vi "Solve_Correspond_Problem_based_on_Cost_F()-4.vi"(0 "[IN] Cost function":i8[](array[numeric]), 1 "[IN] Still connected\ntracks in group":T2, 3 "[IN] Subtracks":T3(array[cluster]), 7 "[IN] Index of Earliest \nProblem Point Inside":i32, 9 "[IN] # of Longest track\nInside the Tracks Group":i32, 11 "error IN":errorcluster, 13 "[IN] Special case!":bool) -> (4 "[OUT] Clusters for Re\nconstructed Tracks":T1, 15 "error OUT":errorcluster)   [LabVIEW 2013]
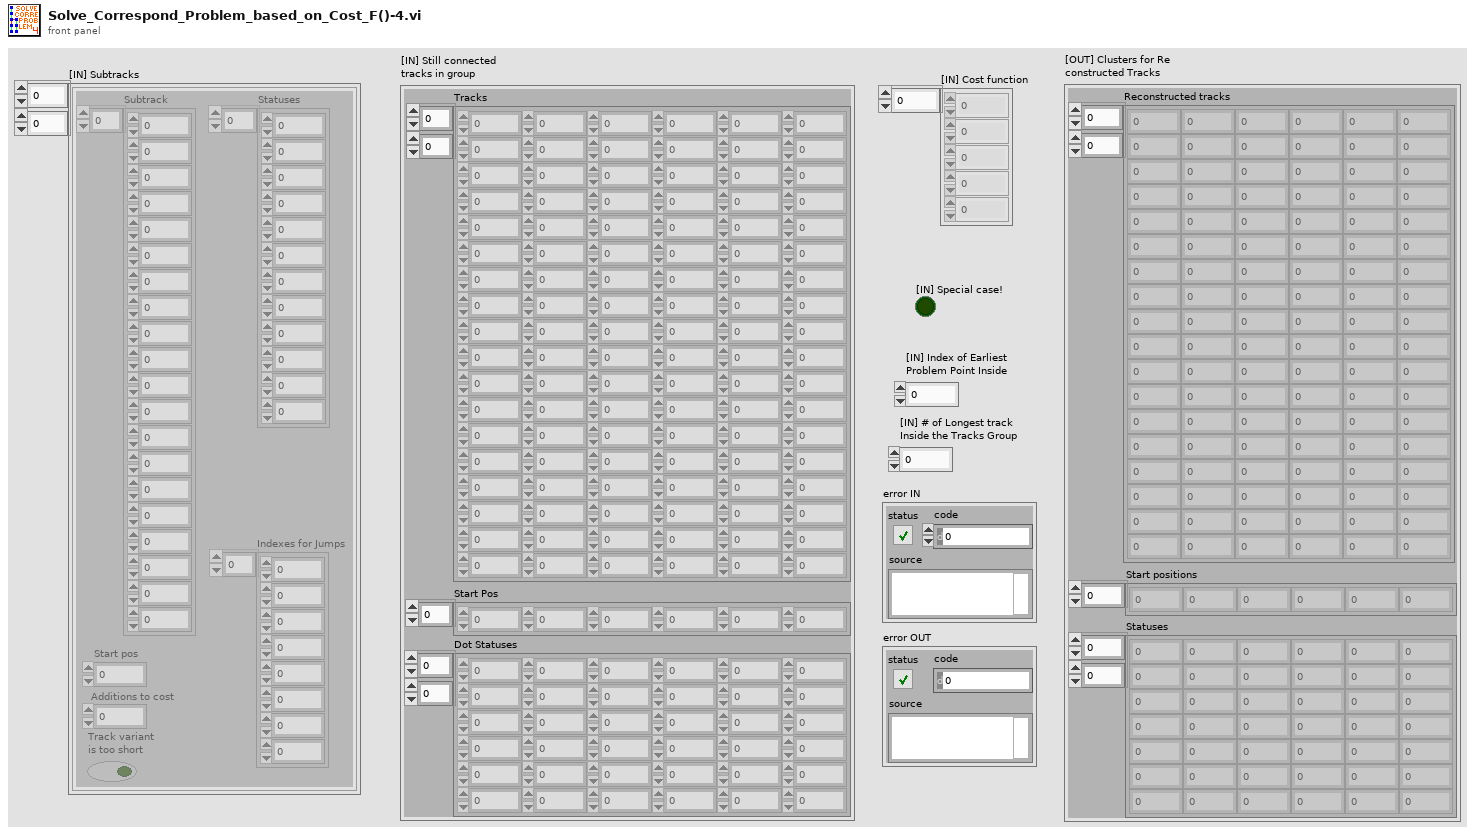
[diagram p1: front panel]
types:
  T1 = cluster{"Reconstructed tracks":dbl[][], "Start positions":i32[], "Statuses":i16[][]}
  T2 = cluster{"Tracks":dbl[][], "Start Pos":i32[], "Dot Statuses":i16[][]}
  T3 = cluster{"Subtrack":dbl[], "Statuses":i16[], "Start pos":i32, "Additions to cost":i32, "Track variant \nis too short":bool, "Indexes for Jumps":i32[]}[][]
  T4 = cluster{"Subtrack":dbl[], "Statuses":i16[], "Start pos":i32, "Additions to cost":i32, "Track variant \nis too short":bool, "Indexes for Jumps":i32[]}
  T5 = cluster{"Subtrack":dbl[], "Statuses":i16[], "Start pos":i32, "Additions to cost":i32, "Track variant \nis too short":bool, "Indexes for Jumps":i32[]}[]
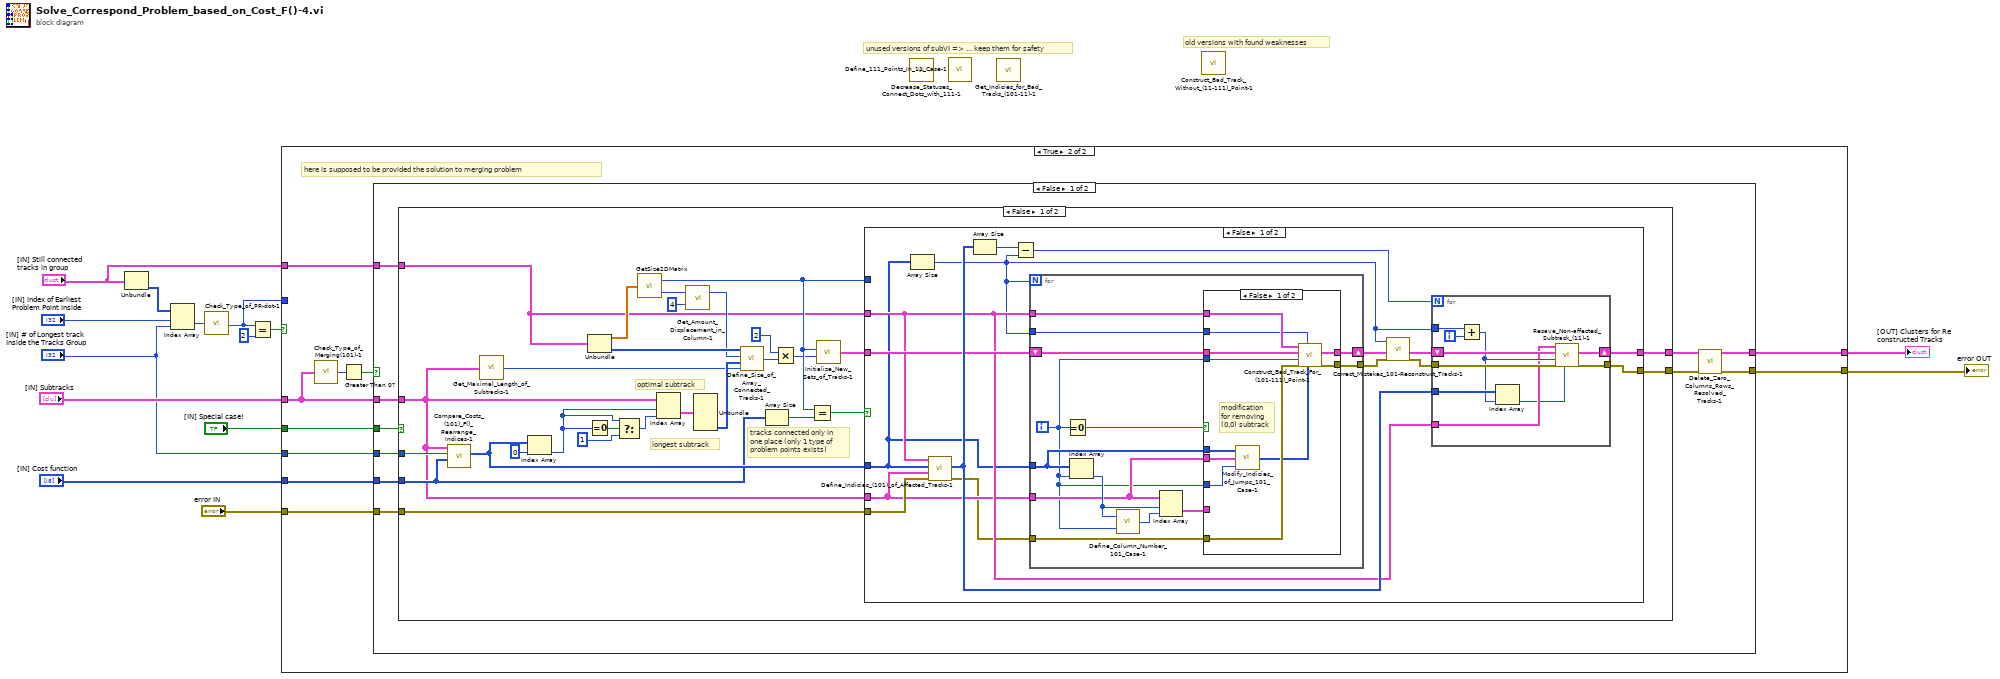
[diagram p0: block diagram]
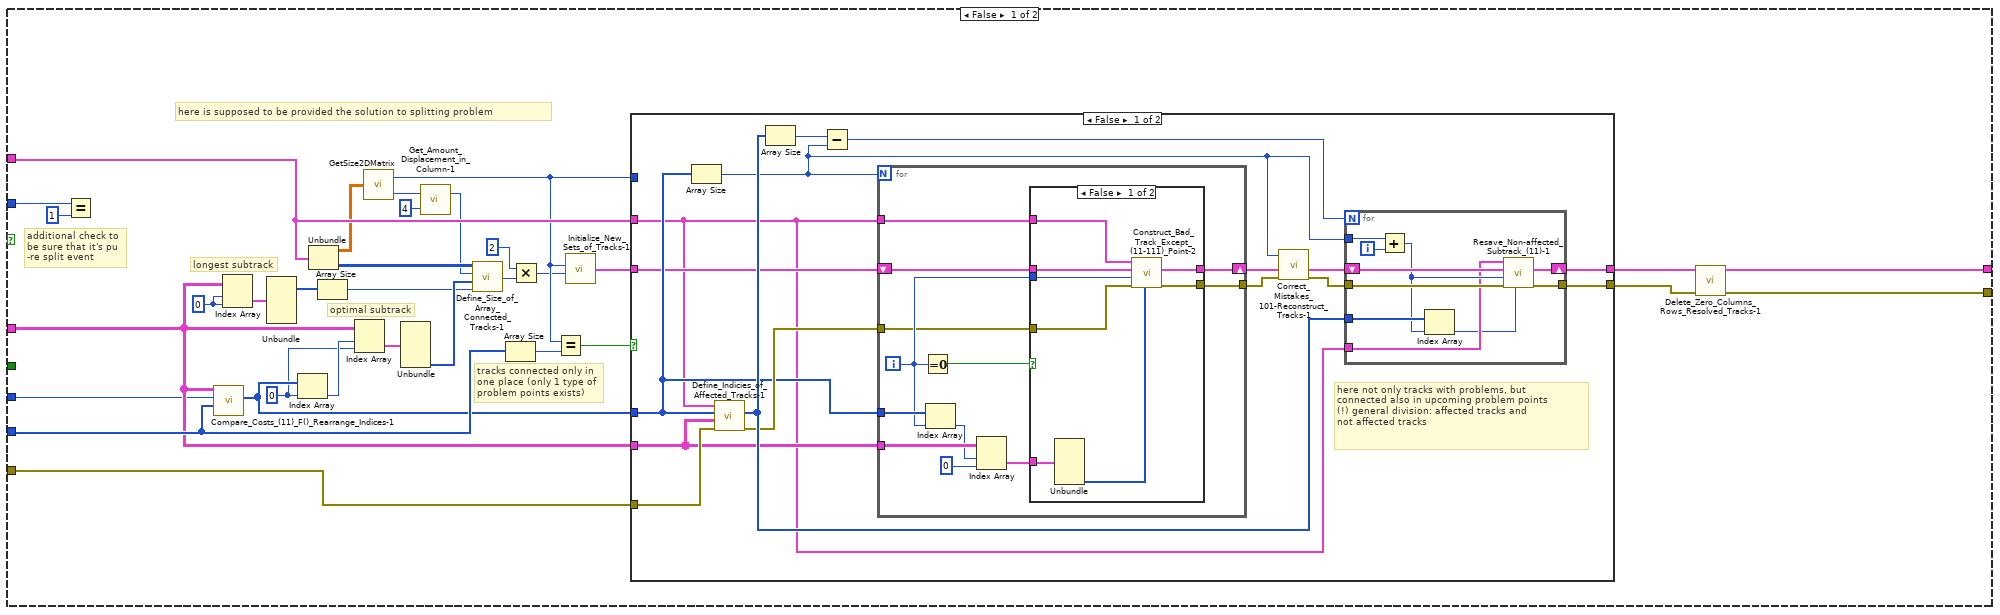
[diagram p2: hidden frame]
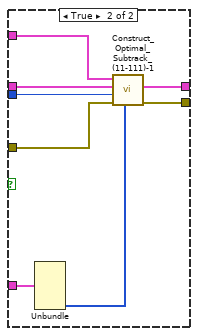
[diagram p3: hidden frame]
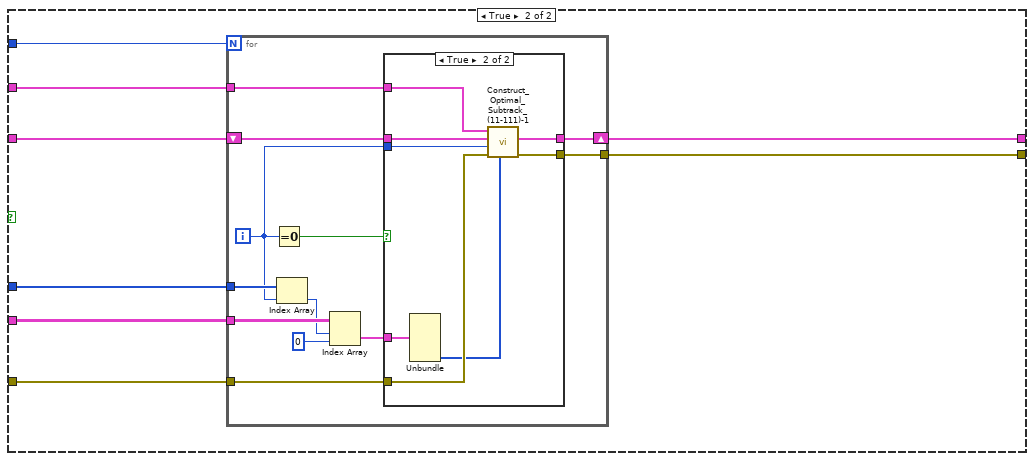
[diagram p4: hidden frame]
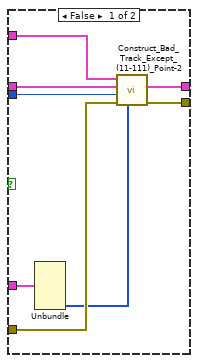
[diagram p5: hidden frame]
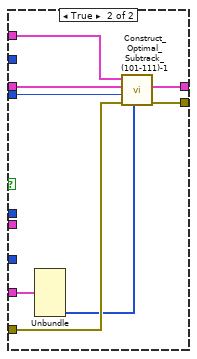
[diagram p6: hidden frame]
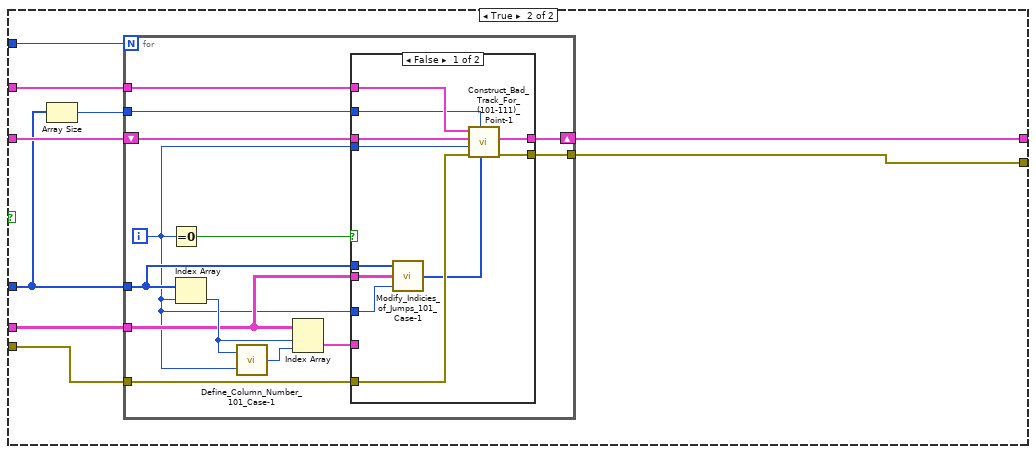
[diagram p7: hidden frame]
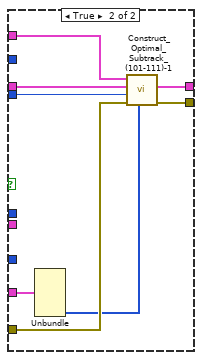
[diagram p8: hidden frame]
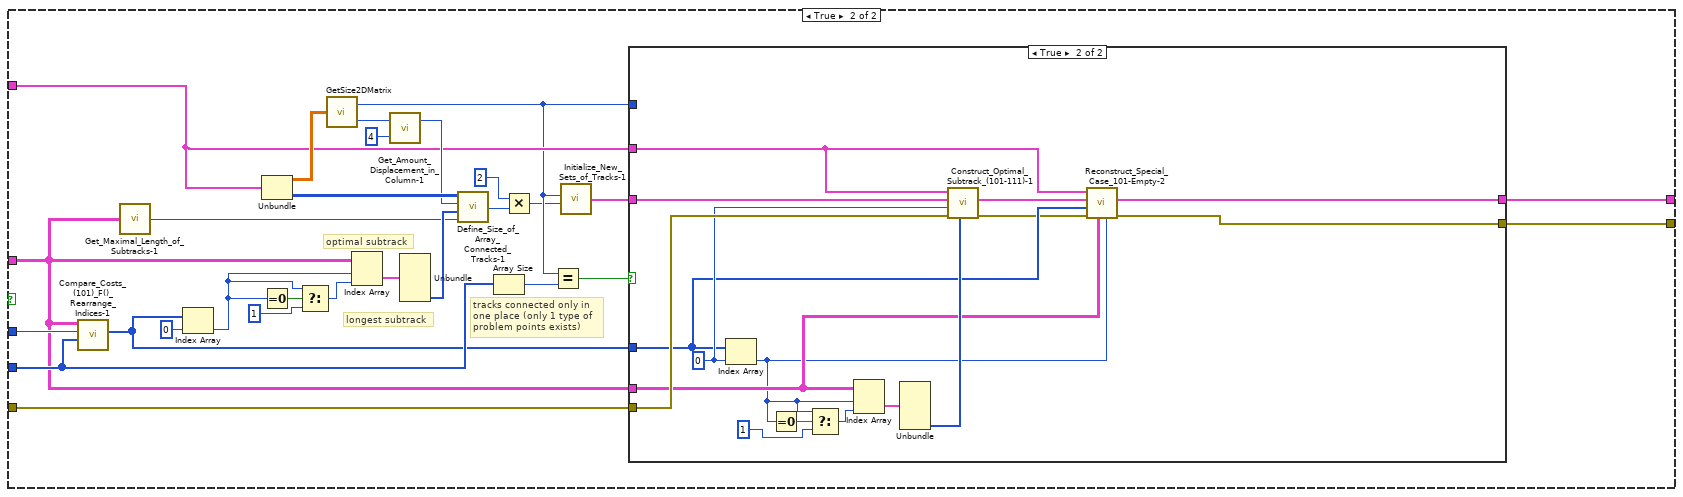
[diagram p9: hidden frame]
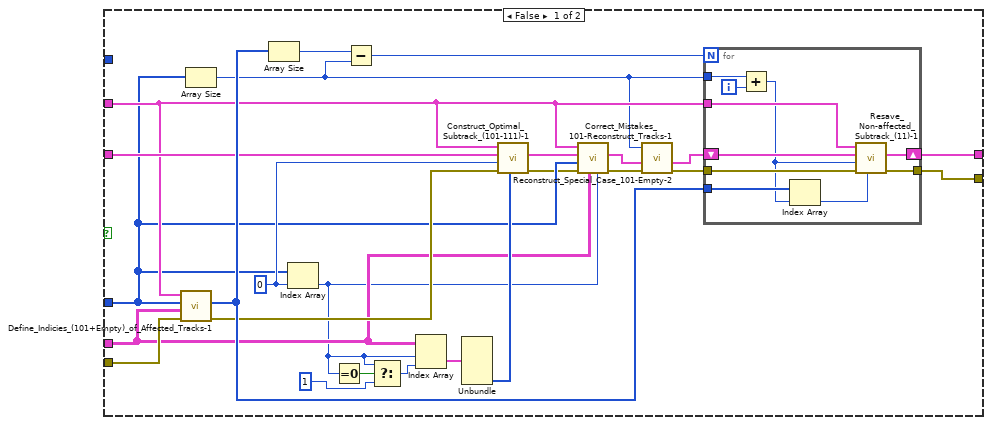
[diagram p10: hidden frame]
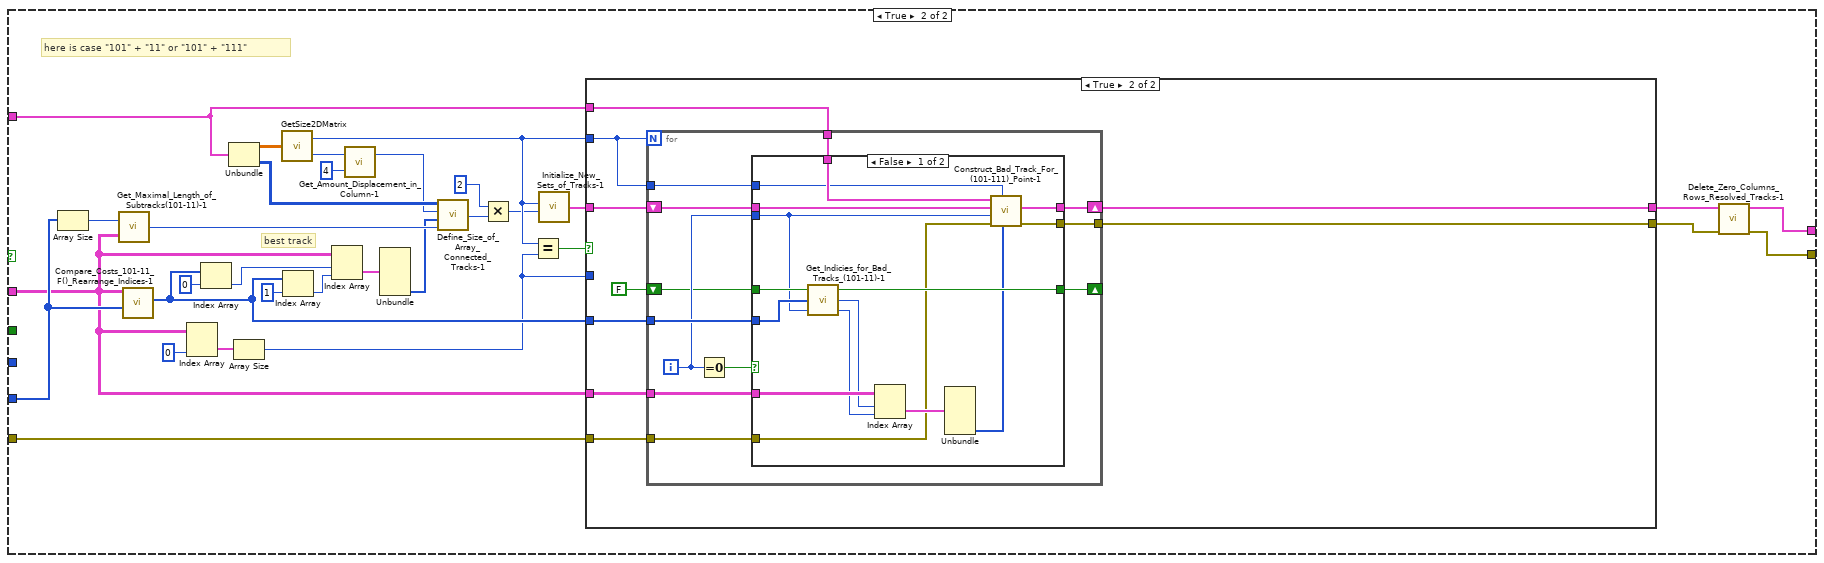
[diagram p11: hidden frame]
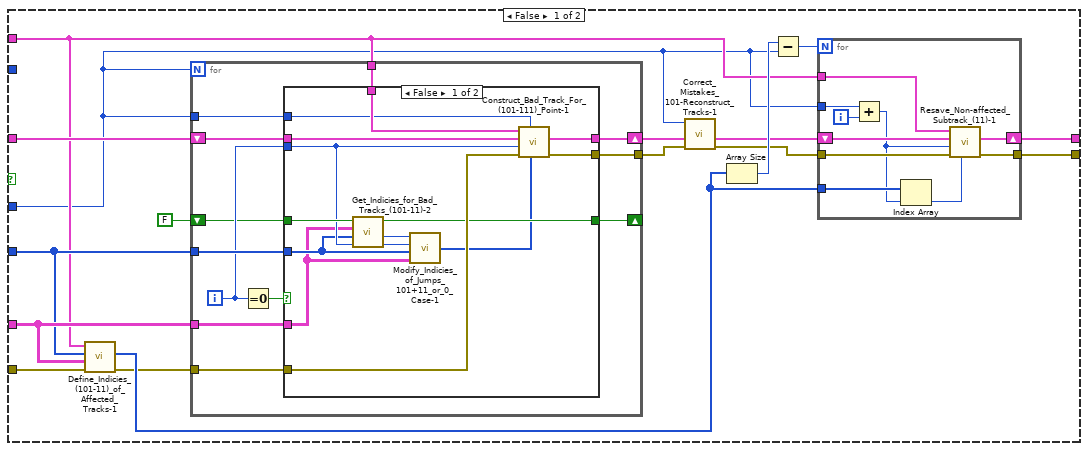
[diagram p12: hidden frame]
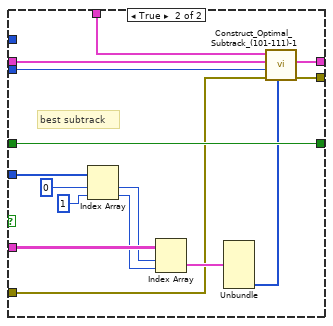
[diagram p13: hidden frame]
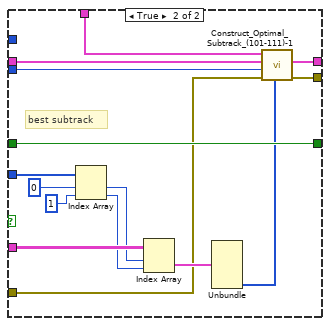
[diagram p14: hidden frame]
diagram:
  # "old versions with found weaknesses"
  # "unused versions of subVI => ... keep them for safety"
  n1 = Unbundle("[IN] Still connected\ntracks in group") -> ("Dot Statuses"=w13:i16[][])  [unwired: 2 out]
  n2 = Index Array(array=w13, index (row)="[IN] Index of Earliest \nProblem Point Inside", index (col)="[IN] # of Longest track\nInside the Tracks Group") -> (element=w12:i16)
  n3 = call "Check_Type_of_PR-dot-1.vi"("[IN] dot status"=w12) -> ("[OUT] Type of\nproblem dot"=w5:i32)
  n4 = Equal?(x=w5, y=2) -> (x = y?=w11:bool)
  n5 = case shown="True" w11 {
    tunnel: "[IN] Subtracks" -> [w45 w141]
    tunnel: "[IN] Still connected\ntracks in group" -> [w42 w145]
    tunnel: "error IN" -> [w40 w146]
    tunnel: "[IN] Cost function" -> [w46 w143]
    tunnel: w5 -> [w44 _]
    tunnel: "[IN] # of Longest track\nInside the Tracks Group" -> [w41 w144]
    tunnel: [w39 w139] -> w3
    tunnel: [w38 w138] -> w2
    tunnel: "[IN] Special case!" -> [_ w137]
    frame False {
      w23 = 0 ("index")
      w29 = 0 ("index")
      # "longest subtrack"
      # "tracks connected only in \none place (only 1 type of \nproblem points exists)"
      # "here is supposed to be provided the solution to splitting problem"
      # "optimal subtrack"
      # "additional check to \nbe sure that it's pu\n-re split event"
      n6 = Equal?(x=w44, y=1) -> ()  [unwired: 1 out]
      n7 = call "Compare_Costs_(11)_F()_Rearrange_Indices-1.vi"("[IN] Cost functions"=w46, "[IN] # of Longest track\nInside the Tracks Group"=w41, "[IN] Subtracks"=w45) -> ("[OUT] Indicies of sub\ntracks for transforma\ntion (resolving)"=w30:i32[])  [unwired: 4 in]
      n8 = Index Array(array=w45, index (row)=w23, index (col)=w23) -> (element=w22:T4)
      n9 = Unbundle(w22) -> ("Statuses"=w21:i16[])  [unwired: 5 out]
      n10 = Index Array(array=w30, index=w29) -> (element=w31:i32)
      n11 = Unbundle(w42) -> ("Tracks"=w34:dbl[][], "Dot Statuses"=w36:i16[][])  [unwired: 1 out]
      n12 = Array Size(array=w21) -> (size(s)=w20:i32)
      n13 = Index Array(array=w45, index (row)=w31, index (col)=w29) -> (element=w37:T4)
      n14 = call "GetSize2DMatrix.vi"("Array IN (2D)"=w34) -> ("# Cols"=w28:i32, "# Rows"=w26:i32)
      n15 = Unbundle(w37) -> ("Indexes for Jumps"=w35:i32[])  [unwired: 5 out]
      n16 = call "Get_Amount_Displacement_in_Column-1.vi"("multiplier"=4, "# Rows"=w26) -> ("Displ amount"=w24:i32)  [unwired: 1 out]
      n17 = call "Define_Size_of_Array_Connected_Tracks-1.vi"("[IN] Size of Longest Array\nbetween Subtracks (0,0)"=w20, "[IN] Indexes for Jumps"=w35, "[IN] Original Array Size"=w24, "[IN] Dot Statuses"=w36) -> ("[OUT] # of Eleme\nnts in new Track"=w17:i32)  [unwired: 2 in]
      n18 = Array Size(array=w46) -> (size(s)=w33:i32)
      n19 = Multiply(x=2, y=w17) -> (x*y=w16:i32)
      n20 = Equal?(x=w28, y=w33) -> (x = y?=w32:bool)
      n21 = call "Initialize_New_Sets_of_Tracks-1.vi"("[IN] # of Eleme\nnts in New Tracks"=w16, "[IN] # previously \nconnected tracks"=w28) -> ("[OUT] Clusters for Re\nconstructed Tracks"=w27:T1)  [unwired: 4 in]
      n22 = case shown="False" w32 {
        tunnel: w28 -> [_ w108]
        tunnel: w42 -> [w52 w103]
        tunnel: w30 -> [w54 w107]
        tunnel: w45 -> [w56 w102]
        tunnel: w27 -> [w53 w106]
        tunnel: w40 -> [w62 w101]
        tunnel: [w57 w104] -> w19
        tunnel: [w58 w105] -> w18
        frame False {
          # "here not only tracks with problems, but\nconnected also in upcoming problem points\n(!) general division: affected tracks and \nnot affected tracks"
          n23 = Array Size(array=w54) -> (size(s)=w50:i32)
          n24 = call "Define_Indicies_of_Affected_Tracks-1.vi"("error IN"=w62, "[IN] Subtracks"=w56, "[IN] Indicies of sub\ntracks for transforma\ntion (resolving)"=w54, "[IN] Still connected\ntracks in group"=w52) -> ("error OUT"=w55:errorcluster, "[OUT] Indicies for Tr-\nack Reconstruction"=w59:i32[])  [unwired: 2 in]
          n25 = Array Size(array=w59) -> (size(s)=w61:i32)
          n26 = Subtract(x=w61, y=w50) -> (x-y=w60:i32)
          n27 = for {
            N: w50 -> [_]
            tunnel: w52 -> [w68]
            tunnel: w54 -> [w73]
            tunnel: w56 -> [w72]
            shift-right: [w65] -> w51
            shift-left: w53 -> [w67]
            tunnel: [w64] -> w48
            tunnel: w55 -> [w63]
            i -> [w66]
            n28 = Equal To 0?(x=w66) -> (x = 0?=w74:bool)
            n29 = Index Array(array=w73, index=w66) -> (element=w71:i32)
            n30 = Index Array(array=w72, index (row)=w71, index (col)=0 ("disabled index (col)")) -> (element=w69:T4)
            n31 = case shown="False" w74 {
              tunnel: w69 -> [w82 w90]
              tunnel: w68 -> [w81 w89]
              tunnel: w67 -> [w80 w87]
              tunnel: w66 -> [w79 w86]
              tunnel: [w75 w84] -> w65
              tunnel: w63 -> [w78 w88]
              tunnel: [w76 w83] -> w64
              frame False {
                n32 = Unbundle(w82) -> ("Indexes for Jumps"=w77:i32[])  [unwired: 5 out]
                n33 = call "Construct_Bad_Track_Except_(11-111)_Point-2.vi"("[IN] Indexes for Jumps"=w77, "error IN"=w78, "[IN] Index of recon\nstructed tracks"=w79, "[IN] Clusters for Re\nconstructed Tracks"=w80, "[IN] Still connected\ntracks in group"=w81) -> ("error OUT"=w76:errorcluster, "[OUT] Clusters for Re\nconstructed Tracks"=w75:T1)  [unwired: 5 in]
              }
              frame True {
                n34 = Unbundle(w90) -> ("Indexes for Jumps"=w85:i32[])  [unwired: 5 out]
                n35 = call "Construct_Optimal_Subtrack_(11-111)-1.vi"("[IN] Indexes for Jumps"=w85, "error IN"=w88, "[IN] Index of recon\nstructed tracks"=w86, "[IN] Clusters for Re\nconstructed Tracks"=w87, "[IN] Still connected\ntracks in group"=w89) -> ("error OUT"=w83:errorcluster, "[OUT] Clusters for Re\nconstructed Tracks"=w84:T1)  [unwired: 5 in]
              }
            }
          }
          n36 = call "Correct_Mistakes_101-Reconstruct_Tracks-1.vi"("error IN"=w48, "[IN] Clusters for Re\nconstructed Tracks"=w51, "[IN] Number of Subtracks"=w50) -> ("error OUT"=w47:errorcluster, "[OUT] Clusters for Re\nconstructed Tracks"=w49:T1)  [unwired: 3 in]
          n37 = for {
            N: w60 -> [_]
            tunnel: w47 -> [w96]
            tunnel: w59 -> [w100]
            tunnel: w50 -> [w98]
            tunnel: w52 -> [w94]
            shift-right: [w92] -> w57
            shift-left: w49 -> [w97]
            tunnel: [w91] -> w58
            i -> [w99]
            n38 = Add(x=w98, y=w99) -> (x+y=w95:i32)
            n39 = Index Array(array=w100, index=w95) -> (element=w93:i32)
            n40 = call "Resave_Non-affected_Subtrack_(11)-1.vi"("[IN] Index for Not\nAffected Track"=w93, "error IN"=w96, "[IN] Index of recon\nstructed tracks"=w95, "[IN] Clusters for Re\nconstructed Tracks"=w97, "[IN] Still connected\ntracks in group"=w94) -> ("error OUT"=w91:errorcluster, "[OUT] Clusters for Re\nconstructed Tracks"=w92:T1)  [unwired: 5 in]
          }
        }
        frame True {
          n41 = for {
            N: w108 -> [_]
            tunnel: w103 -> [w114]
            tunnel: w107 -> [w119]
            tunnel: w102 -> [w118]
            shift-right: [w111] -> w104
            shift-left: w106 -> [w113]
            tunnel: w101 -> [w110]
            tunnel: [w109] -> w105
            i -> [w112]
            n42 = Equal To 0?(x=w112) -> (x = 0?=w120:bool)
            n43 = Index Array(array=w119, index=w112) -> (element=w117:i32)
            n44 = Index Array(array=w118, index (row)=w117, index (col)=0 ("disabled index (col)")) -> (element=w115:T4)
            n45 = case shown="True" w120 {
              tunnel: w115 -> [w128 w136]
              tunnel: w114 -> [w127 w135]
              tunnel: w113 -> [w126 w133]
              tunnel: w112 -> [w125 w132]
              tunnel: [w122 w130] -> w111
              tunnel: w110 -> [w124 w134]
              tunnel: [w121 w129] -> w109
              frame False {
                n46 = Unbundle(w128) -> ("Indexes for Jumps"=w123:i32[])  [unwired: 5 out]
                n47 = call "Construct_Bad_Track_Except_(11-111)_Point-2.vi"("[IN] Indexes for Jumps"=w123, "error IN"=w124, "[IN] Index of recon\nstructed tracks"=w125, "[IN] Clusters for Re\nconstructed Tracks"=w126, "[IN] Still connected\ntracks in group"=w127) -> ("error OUT"=w121:errorcluster, "[OUT] Clusters for Re\nconstructed Tracks"=w122:T1)  [unwired: 5 in]
              }
              frame True {
                n48 = Unbundle(w136) -> ("Indexes for Jumps"=w131:i32[])  [unwired: 5 out]
                n49 = call "Construct_Optimal_Subtrack_(11-111)-1.vi"("[IN] Indexes for Jumps"=w131, "error IN"=w134, "[IN] Index of recon\nstructed tracks"=w132, "[IN] Clusters for Re\nconstructed Tracks"=w133, "[IN] Still connected\ntracks in group"=w135) -> ("error OUT"=w129:errorcluster, "[OUT] Clusters for Re\nconstructed Tracks"=w130:T1)  [unwired: 5 in]
              }
            }
          }
        }
      }
      n50 = call "Delete_Zero_Columns_Rows_Resolved_Tracks-1.vi"("error IN"=w18, "[IN] Clusters for Re\nconstructed Tracks"=w19) -> ("error OUT"=w38:errorcluster, "[OUT] Clusters for Re\nconstructed Tracks"=w39:T1)  [unwired: 4 in]
    }
    frame True {
      # "here is supposed to be provided the solution to merging problem"
      n51 = call "Check_Type_of_Merging(101)-1.vi"("[IN] Subtracks"=w141) -> ("[OUT] # of Additional Costs"=w142:i32)
      n52 = Greater Than 0?(x=w142) -> (x > 0?=w140:bool)
      n53 = case shown="False" w140 {
        tunnel: w146 -> [w156 w372]
        tunnel: w145 -> [w155 w371]
        tunnel: w144 -> [w154 _]
        tunnel: w143 -> [w151 w393]
        tunnel: w141 -> [w150 w373]
        tunnel: [w153 w367] -> w139
        tunnel: [w152 w366] -> w138
        tunnel: w137 -> [w147 _]
        frame False {
          n54 = case shown="False" w147 {
            tunnel: w156 -> [w173 w288]
            tunnel: w155 -> [w172 w292]
            tunnel: w154 -> [w170 w297]
            tunnel: w151 -> [w163 w296]
            tunnel: w150 -> [w162 w287]
            tunnel: [w161 w295] -> w149
            tunnel: [w160 w294] -> w148
            frame False {
              # "longest subtrack"
              # "tracks connected only in \none place (only 1 type of \nproblem points exists)"
              # "optimal subtrack"
              n55 = call "Compare_Costs_(101)_F()_Rearrange_Indices-1.vi"("[IN] Cost functions"=w163, "[IN] # of Longest track\nInside the Tracks Group"=w170, "[IN] Subtracks"=w162) -> ("[OUT] Indicies of sub\ntracks for transforma\ntion (resolving)"=w169:i32[])  [unwired: 4 in]
              n56 = call "Get_Maximal_Length_of_Subtracks-1.vi"("[IN] Subtracks"=w162) -> ("[OUT] Maximal Length"=w171:i32)
              n57 = Index Array(array=w169, index=0) -> (element=w165:i32)
              n58 = Unbundle(w172) -> ("Tracks"=w181:dbl[][], "Dot Statuses"=w183:i16[][])  [unwired: 1 out]
              n59 = Equal To 0?(x=w165) -> (x = 0?=w167:bool)
              n60 = Select(t=w165, s=w167, f=1) -> (s? t:f=w164:i32)
              n61 = call "GetSize2DMatrix.vi"("Array IN (2D)"=w181) -> ("# Cols"=w178:i32, "# Rows"=w176:i32)
              n62 = Index Array(array=w162, index (row)=w165, index (col)=w164) -> (element=w184:T4)
              n63 = call "Get_Amount_Displacement_in_Column-1.vi"("multiplier"=4, "# Rows"=w176) -> ("Displ amount"=w174:i32)  [unwired: 1 out]
              n64 = Unbundle(w184) -> ("Indexes for Jumps"=w182:i32[])  [unwired: 5 out]
              n65 = call "Define_Size_of_Array_Connected_Tracks-1.vi"("[IN] Size of Longest Array\nbetween Subtracks (0,0)"=w171, "[IN] Indexes for Jumps"=w182, "[IN] Original Array Size"=w174, "[IN] Dot Statuses"=w183) -> ("[OUT] # of Eleme\nnts in new Track"=w159:i32)  [unwired: 2 in]
              n66 = Array Size(array=w163) -> (size(s)=w180:i32)
              n67 = Multiply(x=2, y=w159) -> (x*y=w157:i32)
              n68 = Equal?(x=w178, y=w180) -> (x = y?=w179:bool)
              n69 = call "Initialize_New_Sets_of_Tracks-1.vi"("[IN] # of Eleme\nnts in New Tracks"=w157, "[IN] # previously \nconnected tracks"=w178) -> ("[OUT] Clusters for Re\nconstructed Tracks"=w177:T1)  [unwired: 4 in]
              n70 = case shown="False" w179 {
                tunnel: w178 -> [_ w251]
                tunnel: w172 -> [w195 w250]
                tunnel: w169 -> [w192 w246]
                tunnel: w162 -> [w194 w249]
                tunnel: w177 -> [w196 w247]
                tunnel: w173 -> [w198 w248]
                tunnel: [w190 w244] -> w161
                tunnel: [w191 w243] -> w160
                frame False {
                  n71 = Array Size(array=w192) -> (size(s)=w185:i32)
                  n72 = call "Define_Indicies_(101)_of_Affected_Tracks-1.vi"("error IN"=w198, "[IN] Subtracks"=w194, "[IN] Indicies of sub\ntracks for transforma\ntion (resolving)"=w192, "[IN] Still connected\ntracks in group"=w195) -> ("error OUT"=w193:errorcluster, "[OUT] Indicies for Tr-\nack Reconstruction"=w197:i32[])  [unwired: 2 in]
                  n73 = Array Size(array=w197) -> (size(s)=w200:i32)
                  n74 = Subtract(x=w200, y=w185) -> (x-y=w199:i32)
                  n75 = for {
                    N: w185 -> [_]
                    tunnel: w195 -> [w211]
                    tunnel: w192 -> [w203]
                    tunnel: w194 -> [w202]
                    tunnel: w193 -> [w210]
                    shift-right: [w208] -> w189
                    shift-left: w196 -> [w209]
                    tunnel: [w207] -> w187
                    tunnel: w185 -> [w206]
                    i -> [w201]
                    n76 = Equal To 0?(x=w201) -> (x = 0?=w213:bool)
                    n77 = Index Array(array=w203, index=w201) -> (element=w205:i32)
                    n78 = call "Define_Column_Number_101_Case-1.vi"("[IN] Current index"=w201, "[IN] Index of \nSubtrack Row"=w205) -> ("[OUT] Column for subtrack"=w204:i32)
                    n79 = Index Array(array=w202, index (row)=w205, index (col)=w204) -> (element=w212:T4)
                    n80 = case shown="False" w213 {
                      tunnel: w212 -> [_ w232]
                      tunnel: w211 -> [w221 w231]
                      tunnel: w201 -> [w218 w229]
                      tunnel: w210 -> [w217 w228]
                      tunnel: w209 -> [w219 w230]
                      tunnel: [w214 w225] -> w208
                      tunnel: [w215 w226] -> w207
                      tunnel: w206 -> [w220 _]
                      tunnel: w203 -> [w224 _]
                      tunnel: w202 -> [w223 _]
                      tunnel: w201 -> [w222 _]
                      frame False {
                        # "modification\nfor removing\n(0,0) subtrack"
                        n81 = call "Modify_Indicies_of_Jumps_101_Case-1.vi"("[IN] Current Index"=w222, "[IN] Subtracks"=w223, "[IN] Indicies of sub\ntracks for transforma\ntion (resolving)"=w224) -> ("[OUT] Indicies of Jumps"=w216:i32[])  [unwired: 2 in]
                        n82 = call "Construct_Bad_Track_For_(101-111)_Point-1.vi"("[IN] Indexes for Jumps"=w216, "[IN] Number of Co\nnnected Points"=w220, "error IN"=w217, "[IN] Index of recon\nstructed tracks"=w218, "[IN] Clusters for Re\nconstructed Tracks"=w219, "[IN] Still connected\ntracks in group"=w221) -> ("error OUT"=w215:errorcluster, "[OUT] Clusters for Re\nconstructed Tracks"=w214:T1)  [unwired: 4 in]
                      }
                      frame True {
                        n83 = Unbundle(w232) -> ("Indexes for Jumps"=w227:i32[])  [unwired: 5 out]
                        n84 = call "Construct_Optimal_Subtrack_(101-111)-1.vi"("[IN] Indexes for Jumps"=w227, "error IN"=w228, "[IN] Index of recon\nstructed tracks"=w229, "[IN] Clusters for Re\nconstructed Tracks"=w230, "[IN] Still connected\ntracks in group"=w231) -> ("error OUT"=w226:errorcluster, "[OUT] Clusters for Re\nconstructed Tracks"=w225:T1)  [unwired: 5 in]
                      }
                    }
                  }
                  n85 = call "Correct_Mistakes_101-Reconstruct_Tracks-1.vi"("error IN"=w187, "[IN] Clusters for Re\nconstructed Tracks"=w189, "[IN] Number of Subtracks"=w185) -> ("error OUT"=w186:errorcluster, "[OUT] Clusters for Re\nconstructed Tracks"=w188:T1)  [unwired: 3 in]
                  n86 = for {
                    N: w199 -> [_]
                    tunnel: w186 -> [w238]
                    tunnel: w197 -> [w242]
                    tunnel: w185 -> [w240]
                    tunnel: w195 -> [w236]
                    shift-right: [w234] -> w190
                    shift-left: w188 -> [w239]
                    tunnel: [w233] -> w191
                    i -> [w241]
                    n87 = Add(x=w240, y=w241) -> (x+y=w237:i32)
                    n88 = Index Array(array=w242, index=w237) -> (element=w235:i32)
                    n89 = call "Resave_Non-affected_Subtrack_(11)-1.vi"("[IN] Index for Not\nAffected Track"=w235, "error IN"=w238, "[IN] Index of recon\nstructed tracks"=w237, "[IN] Clusters for Re\nconstructed Tracks"=w239, "[IN] Still connected\ntracks in group"=w236) -> ("error OUT"=w233:errorcluster, "[OUT] Clusters for Re\nconstructed Tracks"=w234:T1)  [unwired: 5 in]
                  }
                }
                frame True {
                  n90 = Array Size(array=w246) -> (size(s)=w245:i32)
                  n91 = for {
                    N: w251 -> [_]
                    tunnel: w250 -> [w262]
                    tunnel: w246 -> [w254]
                    tunnel: w249 -> [w253]
                    tunnel: w248 -> [w261]
                    shift-right: [w259] -> w244
                    shift-left: w247 -> [w260]
                    tunnel: [w258] -> w243
                    tunnel: w245 -> [w257]
                    i -> [w252]
                    n92 = Equal To 0?(x=w252) -> (x = 0?=w264:bool)
                    n93 = Index Array(array=w254, index=w252) -> (element=w256:i32)
                    n94 = call "Define_Column_Number_101_Case-1.vi"("[IN] Current index"=w252, "[IN] Index of \nSubtrack Row"=w256) -> ("[OUT] Column for subtrack"=w255:i32)
                    n95 = Index Array(array=w253, index (row)=w256, index (col)=w255) -> (element=w263:T4)
                    n96 = case shown="False" w264 {
                      tunnel: w263 -> [_ w283]
                      tunnel: w262 -> [w272 w279]
                      tunnel: w252 -> [w268 w280]
                      tunnel: w261 -> [w267 w282]
                      tunnel: w260 -> [w270 w281]
                      tunnel: [w269 w278] -> w259
                      tunnel: [w266 w276] -> w258
                      tunnel: w257 -> [w271 _]
                      tunnel: w254 -> [w275 _]
                      tunnel: w253 -> [w274 _]
                      tunnel: w252 -> [w273 _]
                      frame False {
                        n97 = call "Modify_Indicies_of_Jumps_101_Case-1.vi"("[IN] Current Index"=w273, "[IN] Subtracks"=w274, "[IN] Indicies of sub\ntracks for transforma\ntion (resolving)"=w275) -> ("[OUT] Indicies of Jumps"=w265:i32[])  [unwired: 2 in]
                        n98 = call "Construct_Bad_Track_For_(101-111)_Point-1.vi"("[IN] Indexes for Jumps"=w265, "[IN] Number of Co\nnnected Points"=w271, "error IN"=w267, "[IN] Index of recon\nstructed tracks"=w268, "[IN] Clusters for Re\nconstructed Tracks"=w270, "[IN] Still connected\ntracks in group"=w272) -> ("error OUT"=w266:errorcluster, "[OUT] Clusters for Re\nconstructed Tracks"=w269:T1)  [unwired: 4 in]
                      }
                      frame True {
                        n99 = Unbundle(w283) -> ("Indexes for Jumps"=w277:i32[])  [unwired: 5 out]
                        n100 = call "Construct_Optimal_Subtrack_(101-111)-1.vi"("[IN] Indexes for Jumps"=w277, "error IN"=w282, "[IN] Index of recon\nstructed tracks"=w280, "[IN] Clusters for Re\nconstructed Tracks"=w281, "[IN] Still connected\ntracks in group"=w279) -> ("error OUT"=w276:errorcluster, "[OUT] Clusters for Re\nconstructed Tracks"=w278:T1)  [unwired: 5 in]
                      }
                    }
                  }
                }
              }
            }
            frame True {
              # "longest subtrack"
              # "tracks connected only in \none place (only 1 type of \nproblem points exists)"
              # "optimal subtrack"
              n101 = call "Compare_Costs_(101)_F()_Rearrange_Indices-1.vi"("[IN] Cost functions"=w296, "[IN] # of Longest track\nInside the Tracks Group"=w297, "[IN] Subtracks"=w287) -> ("[OUT] Indicies of sub\ntracks for transforma\ntion (resolving)"=w289:i32[])  [unwired: 4 in]
              n102 = call "Get_Maximal_Length_of_Subtracks-1.vi"("[IN] Subtracks"=w287) -> ("[OUT] Maximal Length"=w303:i32)
              n103 = Index Array(array=w289, index=0) -> (element=w299:i32)
              n104 = Unbundle(w292) -> ("Tracks"=w308:dbl[][], "Dot Statuses"=w310:i16[][])  [unwired: 1 out]
              n105 = Equal To 0?(x=w299) -> (x = 0?=w301:bool)
              n106 = Select(t=w299, s=w301, f=1) -> (s? t:f=w298:i32)
              n107 = call "GetSize2DMatrix.vi"("Array IN (2D)"=w308) -> ("# Cols"=w291:i32, "# Rows"=w306:i32)
              n108 = Index Array(array=w287, index (row)=w299, index (col)=w298) -> (element=w311:T4)
              n109 = call "Get_Amount_Displacement_in_Column-1.vi"("multiplier"=4, "# Rows"=w306) -> ("Displ amount"=w304:i32)  [unwired: 1 out]
              n110 = Unbundle(w311) -> ("Indexes for Jumps"=w309:i32[])  [unwired: 5 out]
              n111 = call "Define_Size_of_Array_Connected_Tracks-1.vi"("[IN] Size of Longest Array\nbetween Subtracks (0,0)"=w303, "[IN] Indexes for Jumps"=w309, "[IN] Original Array Size"=w304, "[IN] Dot Statuses"=w310) -> ("[OUT] # of Eleme\nnts in new Track"=w286:i32)  [unwired: 2 in]
              n112 = Array Size(array=w296) -> (size(s)=w307:i32)
              n113 = Multiply(x=2, y=w286) -> (x*y=w285:i32)
              n114 = Equal?(x=w291, y=w307) -> (x = y?=w290:bool)
              n115 = call "Initialize_New_Sets_of_Tracks-1.vi"("[IN] # of Eleme\nnts in New Tracks"=w285, "[IN] # previously \nconnected tracks"=w291) -> ("[OUT] Clusters for Re\nconstructed Tracks"=w293:T1)  [unwired: 4 in]
              n116 = case shown="True" w290 {
                tunnel: w291 -> [_ _]
                tunnel: w292 -> [w322 w354]
                tunnel: w289 -> [w320 w352]
                tunnel: w287 -> [w318 w350]
                tunnel: w293 -> [w326 w356]
                tunnel: w288 -> [w330 w358]
                tunnel: [w335 w347] -> w295
                tunnel: [w336 w348] -> w294
                frame False {
                  w323 = 0 ("index")
                  n117 = call "Define_Indicies_(101+Empty)_of_Affected_Tracks-1.vi"("error IN"=w330, "[IN] Subtracks"=w318, "[IN] Indicies of sub\ntracks for transforma\ntion (resolving)"=w320, "[IN] Still connected\ntracks in group"=w322) -> ("error OUT"=w325:errorcluster, "[OUT] Indicies for Tr-\nack Reconstruction"=w329:i32[])  [unwired: 2 in]
                  n118 = Array Size(array=w320) -> (size(s)=w312:i32)
                  n119 = Array Size(array=w329) -> (size(s)=w328:i32)
                  n120 = Index Array(array=w320, index=w323) -> (element=w317:i32)
                  n121 = Equal To 0?(x=w317) -> (x = 0?=w334:bool)
                  n122 = Subtract(x=w328, y=w312) -> (x-y=w327:i32)
                  n123 = Select(t=w317, s=w334, f=1) -> (s? t:f=w333:i32)
                  n124 = Index Array(array=w318, index (row)=w317, index (col)=w333) -> (element=w332:T4)
                  n125 = Unbundle(w332) -> ("Indexes for Jumps"=w324:i32[])  [unwired: 5 out]
                  n126 = call "Construct_Optimal_Subtrack_(101-111)-1.vi"("[IN] Indexes for Jumps"=w324, "error IN"=w325, "[IN] Index of recon\nstructed tracks"=w323, "[IN] Clusters for Re\nconstructed Tracks"=w326, "[IN] Still connected\ntracks in group"=w322) -> ("error OUT"=w319:errorcluster, "[OUT] Clusters for Re\nconstructed Tracks"=w321:T1)  [unwired: 5 in]
                  n127 = call "Reconstruct_Special_Case_101-Empty-2.vi"("[IN] Index of \nBest Subtrack"=w317, "[IN] Subtracks"=w318, "error IN"=w319, "[IN] Indicies of sub\ntracks for transforma\ntion (resolving)"=w320, "[IN] Clusters for Re\nconstructed Tracks"=w321, "[IN] Still connected\ntracks in group"=w322) -> ("error OUT"=w315:errorcluster, "[OUT] Clusters for Re\nconstructed Tracks"=w316:T1)  [unwired: 4 in]
                  n128 = call "Correct_Mistakes_101-Reconstruct_Tracks-1.vi"("error IN"=w315, "[IN] Clusters for Re\nconstructed Tracks"=w316, "[IN] Number of Subtracks"=w312) -> ("error OUT"=w313:errorcluster, "[OUT] Clusters for Re\nconstructed Tracks"=w314:T1)  [unwired: 3 in]
                  n129 = for {
                    N: w327 -> [_]
                    tunnel: w313 -> [w344]
                    tunnel: w329 -> [w346]
                    tunnel: w322 -> [w343]
                    shift-right: [w341] -> w335
                    shift-left: w314 -> [w345]
                    tunnel: [w340] -> w336
                    tunnel: w312 -> [w338]
                    i -> [w339]
                    n130 = Add(x=w338, y=w339) -> (x+y=w337:i32)
                    n131 = Index Array(array=w346, index=w337) -> (element=w342:i32)
                    n132 = call "Resave_Non-affected_Subtrack_(11)-1.vi"("[IN] Index for Not\nAffected Track"=w342, "error IN"=w344, "[IN] Index of recon\nstructed tracks"=w337, "[IN] Clusters for Re\nconstructed Tracks"=w345, "[IN] Still connected\ntracks in group"=w343) -> ("error OUT"=w340:errorcluster, "[OUT] Clusters for Re\nconstructed Tracks"=w341:T1)  [unwired: 5 in]
                  }
                }
                frame True {
                  w355 = 0 ("index")
                  n133 = Index Array(array=w352, index=w355) -> (element=w349:i32)
                  n134 = Equal To 0?(x=w349) -> (x = 0?=w362:bool)
                  n135 = Select(t=w349, s=w362, f=1) -> (s? t:f=w360:i32)
                  n136 = Index Array(array=w350, index (row)=w349, index (col)=w360) -> (element=w359:T4)
                  n137 = Unbundle(w359) -> ("Indexes for Jumps"=w357:i32[])  [unwired: 5 out]
                  n138 = call "Construct_Optimal_Subtrack_(101-111)-1.vi"("[IN] Indexes for Jumps"=w357, "error IN"=w358, "[IN] Index of recon\nstructed tracks"=w355, "[IN] Clusters for Re\nconstructed Tracks"=w356, "[IN] Still connected\ntracks in group"=w354) -> ("error OUT"=w351:errorcluster, "[OUT] Clusters for Re\nconstructed Tracks"=w353:T1)  [unwired: 5 in]
                  n139 = call "Reconstruct_Special_Case_101-Empty-2.vi"("[IN] Index of \nBest Subtrack"=w349, "[IN] Subtracks"=w350, "error IN"=w351, "[IN] Indicies of sub\ntracks for transforma\ntion (resolving)"=w352, "[IN] Clusters for Re\nconstructed Tracks"=w353, "[IN] Still connected\ntracks in group"=w354) -> ("error OUT"=w348:errorcluster, "[OUT] Clusters for Re\nconstructed Tracks"=w347:T1)  [unwired: 4 in]
                }
              }
            }
          }
          n140 = call "Delete_Zero_Columns_Rows_Resolved_Tracks-1.vi"("error IN"=w148, "[IN] Clusters for Re\nconstructed Tracks"=w149) -> ("error OUT"=w152:errorcluster, "[OUT] Clusters for Re\nconstructed Tracks"=w153:T1)  [unwired: 4 in]
        }
        frame True {
          # "here is case \"101\" + \"11\" or \"101\" + \"111\""
          # "best track"
          n141 = Array Size(array=w393) -> (size(s)=w392:i32)
          n142 = call "Get_Maximal_Length_of_Subtracks(101-11)-1.vi"("[IN] Subtracks"=w373, "[IN] Number of costs"=w392) -> ("[OUT] Maximal Length"=w386:i32)
          n143 = call "Compare_Costs_101-11_F()_Rearrange_Indices-1.vi"("[IN] Cost functions"=w393, "[IN] Subtracks"=w373) -> ("[OUT] Indicies of sub\ntracks for transforma\ntion (resolving)"=w374:i32[])  [unwired: 5 in]
          n144 = Index Array(array=w373, index (col)=0 ("disabled index (col)")) -> (element=w378:T5)  [unwired: 1 in]
          n145 = Index Array(array=w374, index=0) -> (element=w384:i32)
          n146 = Unbundle(w371) -> ("Tracks"=w389:dbl[][], "Dot Statuses"=w388:i16[][])  [unwired: 1 out]
          n147 = Array Size(array=w378) -> (size(s)=w370:i32)
          n148 = call "GetSize2DMatrix.vi"("Array IN (2D)"=w389) -> ("# Cols"=w376:i32, "# Rows"=w391:i32)
          n149 = Index Array(array=w374, index=1) -> (element=w381:i32)
          n150 = Index Array(array=w373, index (row)=w384, index (col)=w381) -> (element=w382:T4)
          n151 = call "Get_Amount_Displacement_in_Column-1.vi"("multiplier"=4, "# Rows"=w391) -> ("Displ amount"=w387:i32)  [unwired: 1 out]
          n152 = Unbundle(w382) -> ("Indexes for Jumps"=w380:i32[])  [unwired: 5 out]
          n153 = call "Define_Size_of_Array_Connected_Tracks-1.vi"("[IN] Size of Longest Array\nbetween Subtracks (0,0)"=w386, "[IN] Indexes for Jumps"=w380, "[IN] Original Array Size"=w387, "[IN] Dot Statuses"=w388) -> ("[OUT] # of Eleme\nnts in new Track"=w365:i32)  [unwired: 2 in]
          n154 = Multiply(x=2, y=w365) -> (x*y=w364:i32)
          n155 = Equal?(x=w376, y=w370) -> (x = y?=w377:bool)
          n156 = call "Initialize_New_Sets_of_Tracks-1.vi"("[IN] # of Eleme\nnts in New Tracks"=w364, "[IN] # previously \nconnected tracks"=w376) -> ("[OUT] Clusters for Re\nconstructed Tracks"=w375:T1)  [unwired: 4 in]
          n157 = case shown="True" w377 {
            tunnel: w376 -> [_ w464]
            tunnel: w375 -> [w404 w467]
            tunnel: w374 -> [w402 w470]
            tunnel: w373 -> [w403 w469]
            tunnel: w372 -> [w410 w468]
            tunnel: w371 -> [w400 w466]
            tunnel: w370 -> [w396 _]
            tunnel: [w406 w463] -> w369
            tunnel: [w405 w462] -> w368
            frame False {
              n158 = call "Define_Indicies_(101-11)_of_Affected_Tracks-1.vi"("error IN"=w410, "[IN] Subtracks"=w403, "[IN] Indicies of sub\ntracks for transforma\ntion (resolving)"=w402, "[IN] Still connected\ntracks in group"=w400) -> ("error OUT"=w401:errorcluster, "[OUT] Indicies for Tr-\nack Reconstruction"=w409:i32[])  [unwired: 2 in]
              n159 = for {
                N: w396 -> [_]
                tunnel: w402 -> [w420]
                tunnel: w403 -> [w421]
                tunnel: w401 -> [w418]
                tunnel: w400 -> [w416]
                shift-right: [w414] -> _
                shift-left: FALSE -> [w415]
                shift-right: [w413] -> w398
                shift-left: w404 -> [w417]
                tunnel: w396 -> [w412]
                tunnel: [w411] -> w397
                i -> [w419]
                n160 = Equal To 0?(x=w419) -> (x = 0?=w422:bool)
                n161 = case shown="False" w422 {
                  tunnel: w421 -> [w424 w451]
                  tunnel: w420 -> [w425 w450]
                  tunnel: w419 -> [w428 w441]
                  tunnel: w418 -> [w436 w440]
                  tunnel: w417 -> [w435 w442]
                  tunnel: w416 -> [w434 w443]
                  tunnel: w415 -> [w430 w444]
                  tunnel: [w429 w444] -> w414
                  tunnel: [w433 w437] -> w413
                  tunnel: w412 -> [w431 _]
                  tunnel: [w432 w438] -> w411
                  frame False {
                    n162 = call "Get_Indicies_for_Bad_Tracks_(101-11)-2.vi"("[IN] Current index"=w428, "[IN] Indicies of subtracks for \ntransformation (resolving)"=w425, "[IN] Subtracks"=w424, "[IN] Competed elonga\ntion is reconstructed?"=w430) -> ("[OUT] Column Number"=w426:i32, "[OUT] Row Number"=w427:i32, "[OUT] Competed elonga\ntion is reconstructed?"=w429:bool)  [unwired: 1 in]
                    n163 = call "Modify_Indicies_of_Jumps_101+11_or_0_Case-1.vi"("[IN] Subtracks"=w424, "[IN] Indicies of sub\ntracks for transforma\ntion (resolving)"=w425, "[IN] Column Number"=w426, "[IN] Row Number"=w427) -> ("[OUT] Indicies of Jumps"=w423:i32[])  [unwired: 2 in]
                    n164 = call "Construct_Bad_Track_For_(101-111)_Point-1.vi"("[IN] Indexes for Jumps"=w423, "[IN] Number of Co\nnnected Points"=w431, "error IN"=w436, "[IN] Index of recon\nstructed tracks"=w428, "[IN] Clusters for Re\nconstructed Tracks"=w435, "[IN] Still connected\ntracks in group"=w434) -> ("error OUT"=w432:errorcluster, "[OUT] Clusters for Re\nconstructed Tracks"=w433:T1)  [unwired: 4 in]
                  }
                  frame True {
                    # "best subtrack"
                    n165 = Index Array(array=w450, index #1=0 ("index"), index #2=1 ("index")) -> (element #1=w447:i32, element #2=w446:i32)
                    n166 = Index Array(array=w451, index (row)=w447, index (col)=w446) -> (element=w445:T4)
                    n167 = Unbundle(w445) -> ("Indexes for Jumps"=w439:i32[])  [unwired: 5 out]
                    n168 = call "Construct_Optimal_Subtrack_(101-111)-1.vi"("[IN] Indexes for Jumps"=w439, "error IN"=w440, "[IN] Index of recon\nstructed tracks"=w441, "[IN] Clusters for Re\nconstructed Tracks"=w442, "[IN] Still connected\ntracks in group"=w443) -> ("error OUT"=w438:errorcluster, "[OUT] Clusters for Re\nconstructed Tracks"=w437:T1)  [unwired: 5 in]
                  }
                }
              }
              n169 = call "Correct_Mistakes_101-Reconstruct_Tracks-1.vi"("error IN"=w397, "[IN] Clusters for Re\nconstructed Tracks"=w398, "[IN] Number of Subtracks"=w396) -> ("error OUT"=w394:errorcluster, "[OUT] Clusters for Re\nconstructed Tracks"=w395:T1)  [unwired: 3 in]
              n170 = Array Size(array=w409) -> (size(s)=w408:i32)
              n171 = Subtract(x=w408, y=w396) -> (x-y=w407:i32)
              n172 = for {
                N: w407 -> [_]
                tunnel: w394 -> [w457]
                tunnel: w409 -> [w461]
                tunnel: w396 -> [w459]
                tunnel: w400 -> [w455]
                shift-right: [w453] -> w406
                shift-left: w395 -> [w458]
                tunnel: [w452] -> w405
                i -> [w460]
                n173 = Add(x=w459, y=w460) -> (x+y=w456:i32)
                n174 = Index Array(array=w461, index=w456) -> (element=w454:i32)
                n175 = call "Resave_Non-affected_Subtrack_(11)-1.vi"("[IN] Index for Not\nAffected Track"=w454, "error IN"=w457, "[IN] Index of recon\nstructed tracks"=w456, "[IN] Clusters for Re\nconstructed Tracks"=w458, "[IN] Still connected\ntracks in group"=w455) -> ("error OUT"=w452:errorcluster, "[OUT] Clusters for Re\nconstructed Tracks"=w453:T1)  [unwired: 5 in]
              }
            }
            frame True {
              n176 = for {
                N: w464 -> [_]
                tunnel: w470 -> [w480]
                tunnel: w469 -> [w481]
                tunnel: w468 -> [w478]
                tunnel: w466 -> [w476]
                shift-right: [w474] -> _
                shift-left: FALSE -> [w475]
                shift-right: [w473] -> w463
                shift-left: w467 -> [w477]
                tunnel: w464 -> [w472]
                tunnel: [w471] -> w462
                i -> [w479]
                n177 = Equal To 0?(x=w479) -> (x = 0?=w482:bool)
                n178 = case shown="False" w482 {
                  tunnel: w481 -> [w494 w512]
                  tunnel: w480 -> [w495 w511]
                  tunnel: w479 -> [w489 w502]
                  tunnel: w478 -> [w490 w501]
                  tunnel: w477 -> [w488 w503]
                  tunnel: w476 -> [w487 w504]
                  tunnel: w475 -> [w497 w505]
                  tunnel: [w496 w505] -> w474
                  tunnel: [w486 w498] -> w473
                  tunnel: w472 -> [w483 _]
                  tunnel: [w485 w499] -> w471
                  frame False {
                    n179 = call "Get_Indicies_for_Bad_Tracks_(101-11)-1.vi"("[IN] Current index"=w489, "[IN] Indicies of subtracks for \ntransformation (resolving)"=w495, "[IN] Competed elonga\ntion is reconstructed?"=w497) -> ("[OUT] Column Number"=w492:i32, "[OUT] Row Number"=w493:i32, "[OUT] Competed elonga\ntion is reconstructed?"=w496:bool)
                    n180 = Index Array(array=w494, index (row)=w493, index (col)=w492) -> (element=w491:T4)
                    n181 = Unbundle(w491) -> ("Indexes for Jumps"=w484:i32[])  [unwired: 5 out]
                    n182 = call "Construct_Bad_Track_For_(101-111)_Point-1.vi"("[IN] Indexes for Jumps"=w484, "[IN] Number of Co\nnnected Points"=w483, "error IN"=w490, "[IN] Index of recon\nstructed tracks"=w489, "[IN] Clusters for Re\nconstructed Tracks"=w488, "[IN] Still connected\ntracks in group"=w487) -> ("error OUT"=w485:errorcluster, "[OUT] Clusters for Re\nconstructed Tracks"=w486:T1)  [unwired: 4 in]
                  }
                  frame True {
                    # "best subtrack"
                    n183 = Index Array(array=w511, index #1=0 ("index"), index #2=1 ("index")) -> (element #1=w508:i32, element #2=w507:i32)
                    n184 = Index Array(array=w512, index (row)=w508, index (col)=w507) -> (element=w506:T4)
                    n185 = Unbundle(w506) -> ("Indexes for Jumps"=w500:i32[])  [unwired: 5 out]
                    n186 = call "Construct_Optimal_Subtrack_(101-111)-1.vi"("[IN] Indexes for Jumps"=w500, "error IN"=w501, "[IN] Index of recon\nstructed tracks"=w502, "[IN] Clusters for Re\nconstructed Tracks"=w503, "[IN] Still connected\ntracks in group"=w504) -> ("error OUT"=w499:errorcluster, "[OUT] Clusters for Re\nconstructed Tracks"=w498:T1)  [unwired: 5 in]
                  }
                }
              }
            }
          }
          n187 = call "Delete_Zero_Columns_Rows_Resolved_Tracks-1.vi"("error IN"=w368, "[IN] Clusters for Re\nconstructed Tracks"=w369) -> ("error OUT"=w366:errorcluster, "[OUT] Clusters for Re\nconstructed Tracks"=w367:T1)  [unwired: 4 in]
        }
      }
    }
  }
  "error OUT" <- w2
  "[OUT] Clusters for Re\nconstructed Tracks" <- w3
  n188 = call "Decrease_Statuses_Connect_Dots_with_111-1.vi"() -> ()  [unwired: 10 in, 2 out]
  n189 = call "Define_111_Points_In_11_Case-1.vi"() -> ()  [unwired: 6 in, 2 out]
  n190 = call "Get_Indicies_for_Bad_Tracks_(101-11)-1.vi"() -> ()  [unwired: 3 in, 3 out]
  n191 = call "Construct_Bad_Track_Without_(11-111)_Point-1.vi"() -> ()  [unwired: 10 in, 2 out]
